vi "Autonomous Independent.vi"   [LabVIEW 2015]
doc: "This VI is called when autonomous begins, and will automatically be terminated when autonomous ends. You can carry out timed or sensor driven robot movement independently without needing to return to the caller."
uses:
  <vilib>/Rock Robotics/WPI/Solenoid/WPI_SolenoidValue.ctl
  <vilib>/Rock Robotics/Network Tables/NT Read String.vi
  <vilib>/Rock Robotics/WPI/Solenoid/WPI_SolenoidSetEnum.vi
  <vilib>/Rock Robotics/WPI/Utilities/WPI_GetSetVariantRefNum.vi
  <vilib>/Rock Robotics/WPI/RobotDrive/WPI_RobotDriveArcadeDrive_Standard(NoSaturation).vi
panel:
  # "Be sure to right-click and choose Data Operations>>Make Current Value default if you want to save the array values with the VI"
types:
  T1 = typedef "WPI_SolenoidValue.ctl" = enum16{"Off", "On", "Forward", "Reverse"}
  T2 = typedef "WPI_SolenoidDevRef.ctl" = cluster{"DevStatus":errorcluster, "Pneumatics Control Module":u8, "Forward Solenoid Channel":T3, "Reverse Solenoid Channel":T3}
  T3 = typedef "WPI_SolenoidChannel.ctl" = enum8{"Solenoid 0", "Solenoid 1", "Solenoid 2", "Solenoid 3", "Solenoid 4", "Solenoid 5", "Solenoid 6", "Solenoid 7", "Invalid"}
  T4 = typedef "WPI_RobotDriveDevRef.ctl" = cluster{"DevStatus":errorcluster, "Motors[]":T5[], "Square Inputs":bool, "Max Output":dbl}
  T5 = typedef "WPI_MotorControlDeviceRef.ctl" = cluster{"DeviceStatus":errorcluster, "Type":T6, "PWM":cluster{"PWM Channel":T7, "DeadBand":T8}, "CAN":cluster{"Device Number":u8, "Control Mode":T9, "Semaphore":T10, "Max Vout":dbl, "TalonSRX Control Mode":T11}, "Invert":bool}
  T6 = typedef "WPI_MotorControlType.ctl" = enum16{"PWM", "CAN", "CANTalonSRX"}
  T7 = typedef "FPGA_DIOPWMChannel.ctl" = enum8{"PWM 0", "PWM 1", "PWM 2", "PWM 3", "PWM 4", "PWM 5", "PWM 6", "PWM 7", "PWM 8", "PWM 9", "PWM MXP 0", "PWM MXP 1", "PWM MXP 2", "PWM MXP 3", "PWM MXP 4", "PWM MXP 5", "PWM MXP 6", "PWM MXP 7", "PWM MXP 8", "PWM MXP 9", "Invalid"}
  T8 = typedef "WPI_PWMDeadband.ctl" = cluster{"Name":string, "maxPositivePwm":i32, "minPositivePwm":i32, "centerPwm":i32, "maxNegativePwm":i32, "minNegativePwm":i32, "angularRange":u16}
  T9 = typedef "WPI_CANJaguar_ControlMode.ctl" = enum8{"Percent VBus", "Current", "Speed", "Position", "Voltage"}
  T10 = typedef "Semaphore RefNum" = refnum<k1>
  T11 = typedef "WPI_CANTalonSRX_APIControlMode.ctl" = enum8{"Percent VBus", "Speed", "Position", "Slave", "Unchanged / Invalid", "Voltage Compensation", "Current", "Motion Profile"}
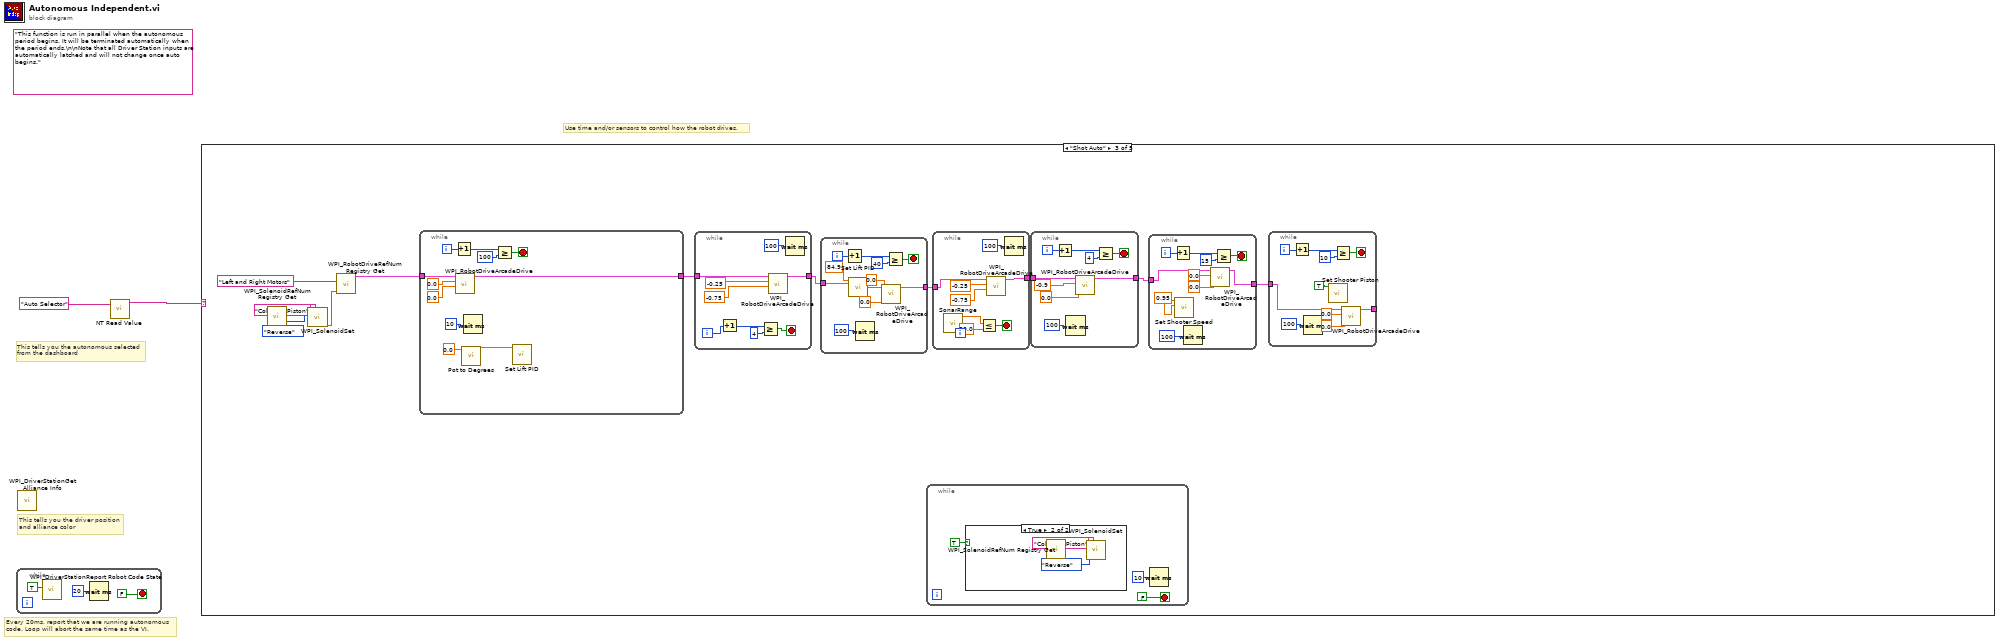
[diagram p0: block diagram]
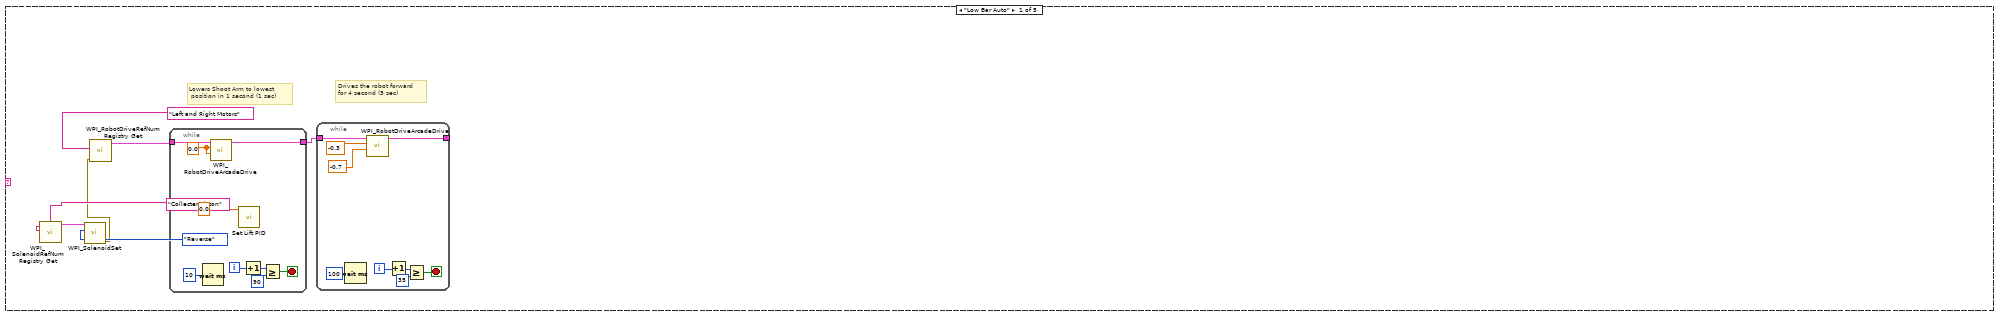
[diagram p2: hidden frame]
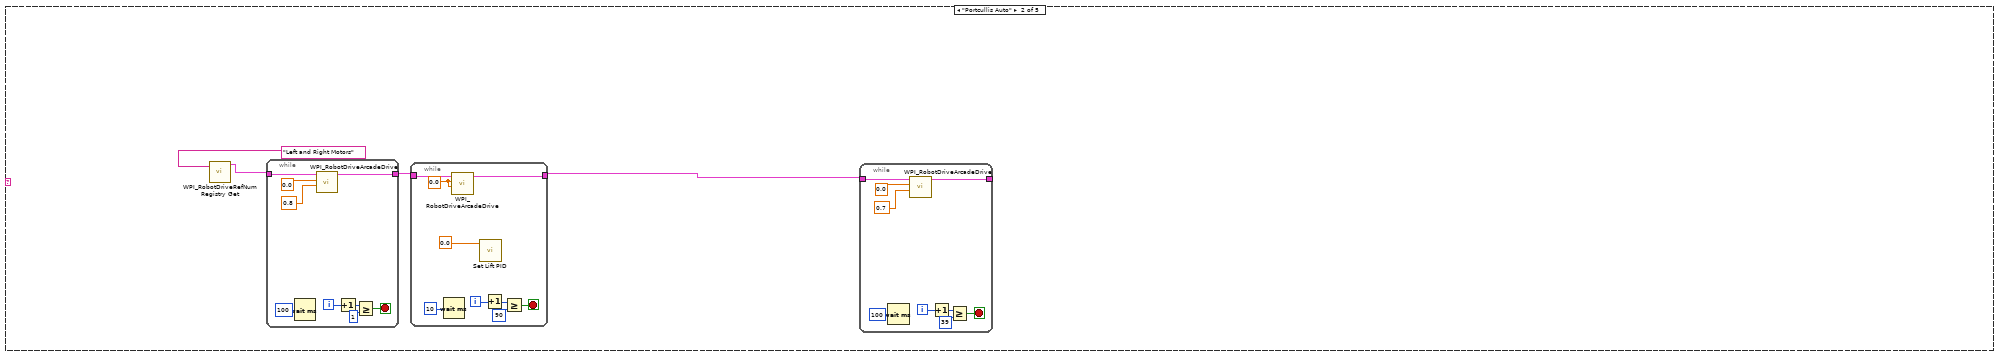
[diagram p3: hidden frame]
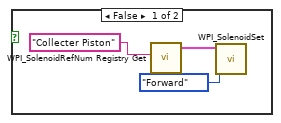
[diagram p4: hidden frame]
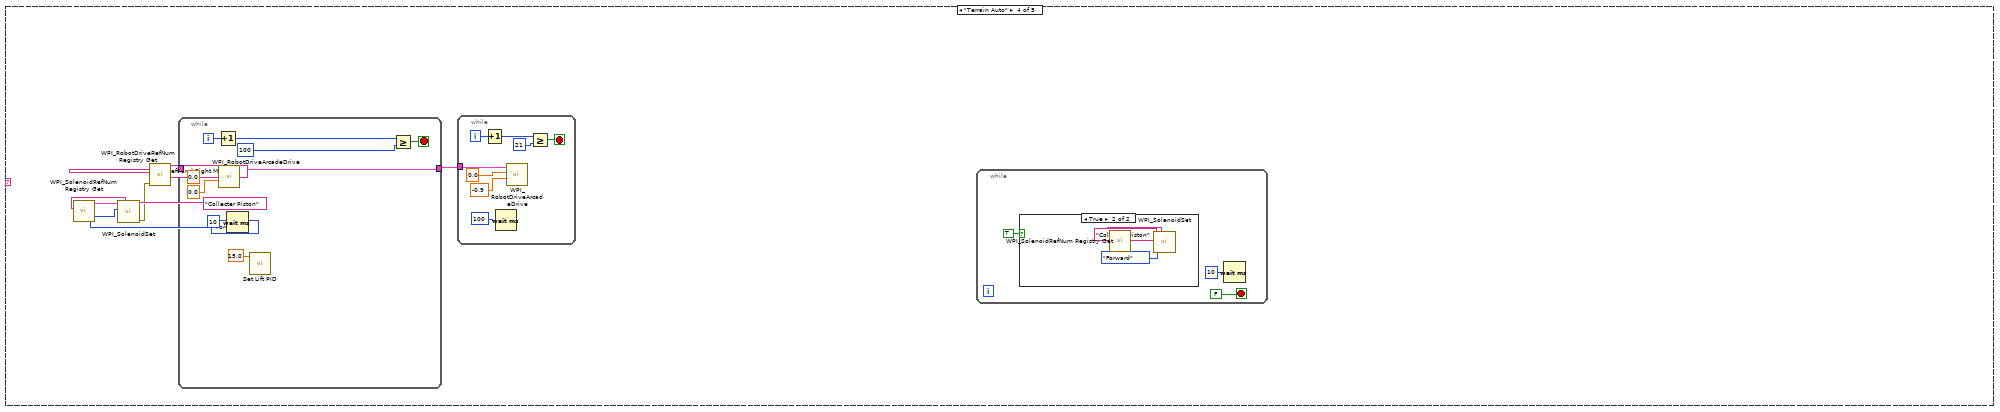
[diagram p5: hidden frame]
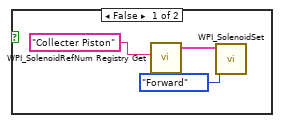
[diagram p6: hidden frame]
diagram:
  (unwired) "This function is run in parallel when the autonomous period begins. It will be terminated automatically when the period ends.\n\nNote that all Driver Station inputs are automatically latched and will not change once auto begins."
  # "This tells you the autonomous selected\nfrom the dashboard"
  # "Every 20ms, report that we are running autonomous\ncode. Loop will abort the same time as the VI."
  # "Use time and/or sensors to control how the robot drives."
  # "This tells you the driver position\nand alliance color"
  n1 = while {
    stop <- FALSE stop-if-true
    n2 = call <vilib>:"WPI_DriverStationReport Robot Code State.vi"("Autonomous"=TRUE) -> ()  [unwired: 10 in, 1 out]
    n3 = Wait (ms)(milliseconds to wait=u32 20) -> ()  [unwired: 1 out]
  }
  n4 = call <vilib>:"WPI_DriverStationGet Alliance Info.vi"() -> ()  [unwired: 12 out]
  n5 = call-poly <vilib>:"NT Read Value.vi"("Name"="Auto Selector") -> ("String"=w1:string)  [unwired: 9 in, 1 out]
  n6 = case shown="\"Shot Auto\"" w1 {
    frame "Low Bar Auto" {
      # "Drives the robot forward\nfor 4 second (5 sec)"
      # "Lowers Shoot Arm to lowest\n position in 1 second (1 sec)"
      n7 = call <vilib>:"WPI_SolenoidRefNum Registry Get.vi"("refnum name"="Collecter Piston") -> ("SolenoidDevRef"=w9:T2)  [unwired: 9 in, 1 out]
      n8 = call-poly <vilib>:"WPI_SolenoidSet.vi"("Value"=WPI_SolenoidValue."Reverse", "SolenoidDevRef"=w9) -> ("error out"=w7:errorcluster)  [unwired: 8 in, 1 out]
      n9 = call <vilib>:"WPI_RobotDriveRefNum Registry Get.vi"("error in (no error)"=w7, "refnum name"="Left and Right Motors") -> ("RobotDriveDevRef"=w11:T4)  [unwired: 8 in, 1 out]
      n10 = while {
        tunnel: w11 -> [w25]
        tunnel: [w24] -> w6
        i -> [w27]
        stop <- w26 stop-if-true
        w23 = 0.0 ("X axis value")
        n11 = Wait (ms)(milliseconds to wait=u32 10) -> ()  [unwired: 1 out]
        n12 = call-poly <vilib>:"WPI_RobotDriveArcadeDrive.vi"("Y axis value"=w23, "X axis value"=w23, "RobotDriveDevRef"=w25) -> ("RobotDriveDevRef"=w24:T4)  [unwired: 6 in, 2 out]
        n13 = call "Set Lift PID.vi"("setpoint"=0.0) -> ()  [unwired: 11 in]
        n14 = Increment(x=w27) -> (x+1=w29:i32)
        n15 = Greater Or Equal?(x=w29, y=90) -> (x >= y?=w26:bool)
      }
      n16 = while {
        tunnel: w6 -> [w14]
        tunnel: [w13] -> _
        i -> [w18]
        stop <- w17 stop-if-true
        n17 = Wait (ms)(milliseconds to wait=u32 100) -> ()  [unwired: 1 out]
        n18 = call-poly <vilib>:"WPI_RobotDriveArcadeDrive.vi"("Y axis value"=-0.7, "X axis value"=-0.3, "RobotDriveDevRef"=w14) -> ("RobotDriveDevRef"=w13:T4)  [unwired: 6 in, 2 out]
        n19 = Increment(x=w18) -> (x+1=w19:i32)
        n20 = Greater Or Equal?(x=w19, y=35) -> (x >= y?=w17:bool)
      }
    }
    frame "Portcullis Auto" {
      n21 = call <vilib>:"WPI_RobotDriveRefNum Registry Get.vi"("refnum name"="Left and Right Motors") -> ("RobotDriveDevRef"=w33:T4)  [unwired: 1 in, 9 out]
      n22 = while {
        tunnel: w33 -> [w54]
        tunnel: [w53] -> w32
        i -> [w58]
        stop <- w57 stop-if-true
        n23 = Wait (ms)(milliseconds to wait=u32 100) -> ()  [unwired: 1 out]
        n24 = call-poly <vilib>:"WPI_RobotDriveArcadeDrive.vi"("Y axis value"=0.8, "X axis value"=0.0, "RobotDriveDevRef"=w54) -> ("RobotDriveDevRef"=w53:T4)  [unwired: 6 in, 2 out]
        n25 = Increment(x=w58) -> (x+1=w59:i32)
        n26 = Greater Or Equal?(x=w59, y=1) -> (x >= y?=w57:bool)
      }
      n27 = while {
        tunnel: w32 -> [w38]
        tunnel: [w37] -> w31
        i -> [w40]
        stop <- w39 stop-if-true
        w36 = 0.0 ("X axis value")
        n28 = Wait (ms)(milliseconds to wait=u32 10) -> ()  [unwired: 1 out]
        n29 = call-poly <vilib>:"WPI_RobotDriveArcadeDrive.vi"("Y axis value"=w36, "X axis value"=w36, "RobotDriveDevRef"=w38) -> ("RobotDriveDevRef"=w37:T4)  [unwired: 6 in, 2 out]
        n30 = call "Set Lift PID.vi"("setpoint"=0.0) -> ()  [unwired: 11 in]
        n31 = Increment(x=w40) -> (x+1=w42:i32)
        n32 = Greater Or Equal?(x=w42, y=90) -> (x >= y?=w39:bool)
      }
      n33 = while {
        tunnel: w31 -> [w45]
        tunnel: [w44] -> _
        i -> [w49]
        stop <- w48 stop-if-true
        n34 = Wait (ms)(milliseconds to wait=u32 100) -> ()  [unwired: 1 out]
        n35 = call-poly <vilib>:"WPI_RobotDriveArcadeDrive.vi"("Y axis value"=0.7, "X axis value"=0.0, "RobotDriveDevRef"=w45) -> ("RobotDriveDevRef"=w44:T4)  [unwired: 6 in, 2 out]
        n36 = Increment(x=w49) -> (x+1=w50:i32)
        n37 = Greater Or Equal?(x=w50, y=39) -> (x >= y?=w48:bool)
      }
    }
    frame "Shot Auto" {
      n38 = call <vilib>:"WPI_SolenoidRefNum Registry Get.vi"("refnum name"="Collecter Piston") -> ("SolenoidDevRef"=w70:T2)  [unwired: 9 in, 1 out]
      n39 = call-poly <vilib>:"WPI_SolenoidSet.vi"("Value"=WPI_SolenoidValue."Reverse", "SolenoidDevRef"=w70) -> ("error out"=w68:errorcluster)  [unwired: 8 in, 1 out]
      n40 = call <vilib>:"WPI_RobotDriveRefNum Registry Get.vi"("error in (no error)"=w68, "refnum name"="Left and Right Motors") -> ("RobotDriveDevRef"=w72:T4)  [unwired: 9 out]
      n41 = while {
        tunnel: w72 -> [w135]
        tunnel: [w134] -> w65
        i -> [w138]
        stop <- w131 stop-if-true
        n42 = Increment(x=w138) -> (x+1=w140:i32)
        n43 = call-poly <vilib>:"WPI_RobotDriveArcadeDrive.vi"("Y axis value"=0.0, "X axis value"=0.0, "RobotDriveDevRef"=w135) -> ("RobotDriveDevRef"=w134:T4)  [unwired: 6 in, 2 out]
        n44 = call "Pot to Degrees.vi"("Pot Value"=0.0 ("setpoint")) -> ("Degrees"=w132:dbl)  [unwired: 10 in]
        n45 = Wait (ms)(milliseconds to wait=u32 10) -> ()  [unwired: 1 out]
        n46 = Greater Or Equal?(x=w140, y=100) -> (x >= y?=w131:bool)
        n47 = call "Set Lift PID.vi"("setpoint"=w132) -> ()  [unwired: 11 in]
      }
      n48 = while {
        tunnel: w65 -> [w81]
        tunnel: [w79] -> w63
        i -> [w75]
        stop <- w74 stop-if-true
        n49 = Increment(x=w75) -> (x+1=w76:i32)
        n50 = Greater Or Equal?(x=w76, y=4) -> (x >= y?=w74:bool)
        n51 = call-poly <vilib>:"WPI_RobotDriveArcadeDrive.vi"("Y axis value"=-0.75, "X axis value"=-0.25, "RobotDriveDevRef"=w81) -> ("RobotDriveDevRef"=w79:T4)  [unwired: 6 in, 2 out]
        n52 = Wait (ms)(milliseconds to wait=u32 100) -> ()  [unwired: 1 out]
      }
      n53 = while {
        tunnel: w63 -> [w104]
        tunnel: [w103] -> w64
        i -> [w111]
        stop <- w110 stop-if-true
        n54 = Increment(x=w111) -> (x+1=w112:i32)
        n55 = call "Set Lift PID.vi"("setpoint"=84.9) -> ()  [unwired: 11 in]
        n56 = Wait (ms)(milliseconds to wait=u32 100) -> ()  [unwired: 1 out]
        n57 = call-poly <vilib>:"WPI_RobotDriveArcadeDrive.vi"("Y axis value"=0.0, "X axis value"=0.0, "RobotDriveDevRef"=w104) -> ("RobotDriveDevRef"=w103:T4)  [unwired: 6 in, 2 out]
        n58 = Greater Or Equal?(x=w112, y=40) -> (x >= y?=w110:bool)
      }
      n59 = while {
        stop <- FALSE stop-if-true
        n60 = case shown="True" TRUE {
          frame False {
            n61 = call <vilib>:"WPI_SolenoidRefNum Registry Get.vi"("refnum name"="Collecter Piston") -> ("SolenoidDevRef"=w126:T2)  [unwired: 9 in, 1 out]
            n62 = call-poly <vilib>:"WPI_SolenoidSet.vi"("Value"=WPI_SolenoidValue."Forward", "SolenoidDevRef"=w126) -> ()  [unwired: 8 in, 2 out]
          }
          frame True {
            n63 = call <vilib>:"WPI_SolenoidRefNum Registry Get.vi"("refnum name"="Collecter Piston") -> ("SolenoidDevRef"=w129:T2)  [unwired: 9 in, 1 out]
            n64 = call-poly <vilib>:"WPI_SolenoidSet.vi"("Value"=WPI_SolenoidValue."Reverse", "SolenoidDevRef"=w129) -> ()  [unwired: 8 in, 2 out]
          }
        }
        n65 = Wait (ms)(milliseconds to wait=u32 10) -> ()  [unwired: 1 out]
      }
      n66 = while {
        tunnel: [w147] -> w67
        tunnel: w64 -> [w142]
        stop <- w145 stop-if-true
        n67 = call "SonarRange.vi"() -> ("Distance"=w143:dbl)  [unwired: 11 in]
        n68 = Less Or Equal?(x=w143, y=80.0) -> (x <= y?=w145:bool)
        n69 = call-poly <vilib>:"WPI_RobotDriveArcadeDrive.vi"("Y axis value"=-0.75, "X axis value"=-0.25, "RobotDriveDevRef"=w142) -> ("RobotDriveDevRef"=w147:T4)  [unwired: 6 in, 2 out]
        n70 = Wait (ms)(milliseconds to wait=u32 100) -> ()  [unwired: 1 out]
      }
      n71 = while {
        tunnel: w67 -> [w120]
        tunnel: [w113] -> w62
        i -> [w118]
        stop <- w117 stop-if-true
        n72 = Increment(x=w118) -> (x+1=w119:i32)
        n73 = Wait (ms)(milliseconds to wait=u32 100) -> ()  [unwired: 1 out]
        n74 = call-poly <vilib>:"WPI_RobotDriveArcadeDrive.vi"("Y axis value"=0.0, "X axis value"=-0.9, "RobotDriveDevRef"=w120) -> ("RobotDriveDevRef"=w113:T4)  [unwired: 6 in, 2 out]
        n75 = Greater Or Equal?(x=w119, y=4) -> (x >= y?=w117:bool)
      }
      n76 = while {
        tunnel: w62 -> [w86]
        tunnel: [w85] -> w66
        i -> [w91]
        stop <- w90 stop-if-true
        w88 = 0.95 ("Set Top Speed")
        n77 = Increment(x=w91) -> (x+1=w92:i32)
        n78 = call "Set Shooter Speed.vi"("Set Bottom Speed"=w88, "Set Top Speed"=w88) -> ()  [unwired: 10 in]
        n79 = Wait (ms)(milliseconds to wait=u32 100) -> ()  [unwired: 1 out]
        n80 = call-poly <vilib>:"WPI_RobotDriveArcadeDrive.vi"("Y axis value"=0.0, "X axis value"=0.0, "RobotDriveDevRef"=w86) -> ("RobotDriveDevRef"=w85:T4)  [unwired: 6 in, 2 out]
        n81 = Greater Or Equal?(x=w92, y=15) -> (x >= y?=w90:bool)
      }
      n82 = while {
        tunnel: w66 -> [w96]
        tunnel: [w93] -> _
        i -> [w101]
        stop <- w100 stop-if-true
        n83 = Increment(x=w101) -> (x+1=w102:i32)
        n84 = Wait (ms)(milliseconds to wait=u32 100) -> ()  [unwired: 1 out]
        n85 = call "Set Shooter Piston.vi"("fire"=TRUE) -> ()  [unwired: 11 in]
        n86 = Greater Or Equal?(x=w102, y=10) -> (x >= y?=w100:bool)
        n87 = call-poly <vilib>:"WPI_RobotDriveArcadeDrive.vi"("Y axis value"=0.0, "X axis value"=0.0, "RobotDriveDevRef"=w96) -> ("RobotDriveDevRef"=w93:T4)  [unwired: 6 in, 2 out]
      }
    }
    frame "Terrain Auto" {
      n88 = call <vilib>:"WPI_SolenoidRefNum Registry Get.vi"("refnum name"="Collecter Piston") -> ("SolenoidDevRef"=w152:T2)  [unwired: 9 in, 1 out]
      n89 = call-poly <vilib>:"WPI_SolenoidSet.vi"("Value"=WPI_SolenoidValue."Forward", "SolenoidDevRef"=w152) -> ("error out"=w150:errorcluster)  [unwired: 8 in, 1 out]
      n90 = call <vilib>:"WPI_RobotDriveRefNum Registry Get.vi"("error in (no error)"=w150, "refnum name"="Left and Right Motors") -> ("RobotDriveDevRef"=w155:T4)  [unwired: 9 out]
      n91 = while {
        tunnel: w155 -> [w169]
        tunnel: [w168] -> w154
        i -> [w172]
        stop <- w167 stop-if-true
        n92 = Increment(x=w172) -> (x+1=w174:i32)
        n93 = call-poly <vilib>:"WPI_RobotDriveArcadeDrive.vi"("Y axis value"=0.0, "X axis value"=0.0, "RobotDriveDevRef"=w169) -> ("RobotDriveDevRef"=w168:T4)  [unwired: 6 in, 2 out]
        n94 = Wait (ms)(milliseconds to wait=u32 10) -> ()  [unwired: 1 out]
        n95 = call "Set Lift PID.vi"("setpoint"=15.0) -> ()  [unwired: 11 in]
        n96 = Greater Or Equal?(x=w174, y=100) -> (x >= y?=w167:bool)
      }
      n97 = while {
        tunnel: w154 -> [w181]
        i -> [w179]
        stop <- w178 stop-if-true
        n98 = Increment(x=w179) -> (x+1=w180:i32)
        n99 = Wait (ms)(milliseconds to wait=u32 100) -> ()  [unwired: 1 out]
        n100 = call-poly <vilib>:"WPI_RobotDriveArcadeDrive.vi"("Y axis value"=-0.9, "X axis value"=0.0, "RobotDriveDevRef"=w181) -> ()  [unwired: 6 in, 3 out]
        n101 = Greater Or Equal?(x=w180, y=21) -> (x >= y?=w178:bool)
      }
      n102 = while {
        stop <- FALSE stop-if-true
        n103 = case shown="True" TRUE {
          frame False {
            n104 = call <vilib>:"WPI_SolenoidRefNum Registry Get.vi"("refnum name"="Collecter Piston") -> ("SolenoidDevRef"=w161:T2)  [unwired: 9 in, 1 out]
            n105 = call-poly <vilib>:"WPI_SolenoidSet.vi"("Value"=WPI_SolenoidValue."Forward", "SolenoidDevRef"=w161) -> ()  [unwired: 8 in, 2 out]
          }
          frame True {
            n106 = call <vilib>:"WPI_SolenoidRefNum Registry Get.vi"("refnum name"="Collecter Piston") -> ("SolenoidDevRef"=w164:T2)  [unwired: 9 in, 1 out]
            n107 = call-poly <vilib>:"WPI_SolenoidSet.vi"("Value"=WPI_SolenoidValue."Forward", "SolenoidDevRef"=w164) -> ()  [unwired: 8 in, 2 out]
          }
        }
        n108 = Wait (ms)(milliseconds to wait=u32 10) -> ()  [unwired: 1 out]
      }
    }
    frame "Do Nothing", Default {
    }
  }
